vi "MFLI--reader--V3.vi"() -> ()   [LabVIEW 2018]
uses:
  publisher action.ctl
  MFLI frontend action.ctl
  mfli reader event.ctl
panel:
  in  "stop  !":bool
  in  "start  !":bool
  in  "set amp! :m":bool
  in  "amplitude (V)":dbl=0.01
  in  "all":enum32{"all"}(tab)
  out "read Voltage (V)":cdb=-2.6434832298996336e-07+7.155979121852138e-05i format="%#10_10f"
  in  "read status":bool
  out "read Voltage X (V)":dbl=-2.6434832298996336e-07 format="%#11_11f"
  out "read Voltage Y (V)":dbl=7.155979121852138e-05 format="%#11_11f"
  in  "delay-read (msec)":i64=200
  out "zi freq (Hz)":dbl=99999.99999990905 format="%-#.3f"
  in  "MFLI Address":string="http://mf-dev4307.local:8004"
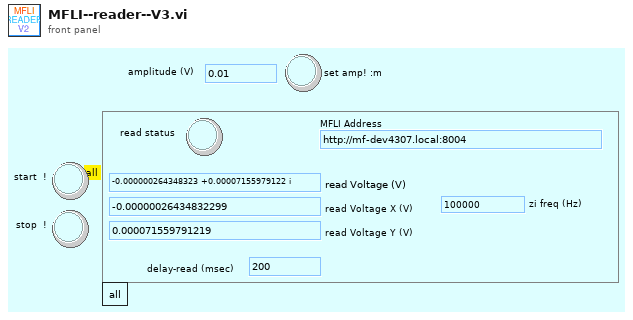
[diagram p1: front panel]
types:
  T1 = typedef "MFLI frontend action.ctl" = enum16{"read", "writeread", "open", "close", "write"}
  T2 = typedef "mfli reader event.ctl" = enum16{"start", "stop"}
  T3 = typedef "publisher action.ctl" = enum16{"set", "get", "init", "check"}
  T4 = typedef "Zurich Instruments LabOne.lvlib/ziTypeHandle.ctl" = cluster{"handleValid":bool, "Conn":u64, "Path Prefix":string, "Handle":u64, "Connected":bool, "Clockbase(s)":dbl}
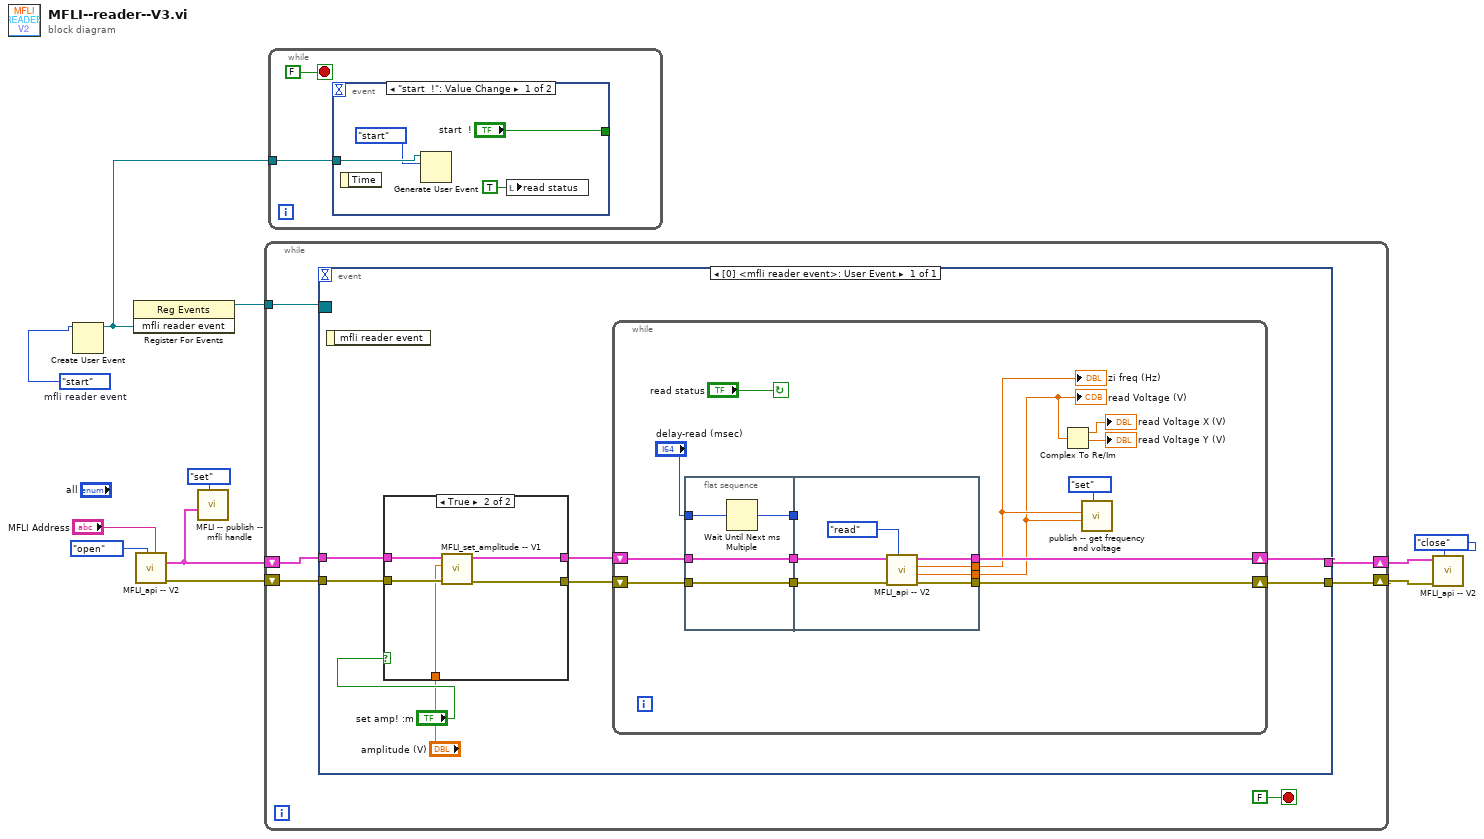
[diagram p0: block diagram]
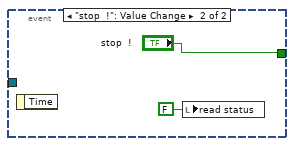
[diagram p3: hidden frame]
diagram:
  w7 = mfli_reader_event."start"  # mfli reader event
  n1 = Create User Event(user event datatype=w7) -> (user event=w6:refnum<user-event>)  [unwired: 1 in, 1 out]
  n2 = register-events(w6) -> (reference out=w8:refnum<event-registration>)  [unwired: 2 in, 1 out]
  n3 = call "MFLI_api -- V2.vi"("MFLI Address"="MFLI Address", "MFLI frontend action"=MFLI_frontend_action."open") -> ("Error Out"=w1:errorcluster, "Handle Out"=w2:T4)  [unwired: 6 in, 2 out]
  n4 = call "MFLI -- publish -- mfli handle.vi"("publisher action"=publisher_action."set", "Handle IN"=w2) -> ()  [unwired: 9 in, 1 out]
  n5 = while {
    tunnel: w8 -> [w17]
    shift-right: [w15] -> w3
    shift-left: w2 -> [w14]
    shift-right: [w16] -> w4
    shift-left: w1 -> [w13]
    stop <- FALSE stop-if-true
    n6 = event shown="[0] <mfli reader event>: User Event" {
      selector: w17 -> [_]
      dyn-events: _ -> [_]
      timeout: _ -> [_]
      tunnel: w14 -> [w24]
      tunnel: w13 -> [w22]
      tunnel: [w19] -> w16
      tunnel: [w18] -> w15
      event User Event {
        n7 = event-data() -> ()  [unwired: 1 in, 1 out]
        n8 = case shown="True" "set amp! :m" {
          tunnel: w24 -> [w27 w32]
          tunnel: [w27 w31] -> w23
          tunnel: w22 -> [w26 w30]
          tunnel: [w26 w29] -> w21
          tunnel: "amplitude (V)" -> [_ w28]
          frame False {
          }
          frame True {
            n9 = call "MFLI_set_amplitude -- V1.vi"("Error In"=w30, "Amp in (V)"=w28, "Handle In"=w32) -> ("Error Out"=w29:errorcluster, "Handle Out"=w31:T4)  [unwired: 5 in, 2 out]
          }
        }
        n10 = while {
          shift-right: [w45] -> w19
          shift-left: w21 -> [w46]
          shift-right: [w43] -> w18
          shift-left: w23 -> [w44]
          stop <- "read status" continue-if-true
          n11 = flat-sequence {
            tunnel: [w50] -> w41
            tunnel: "delay-read (msec)" -> [w49]
            tunnel: [w48] -> w40
            tunnel: w46 -> [w48]
            tunnel: w44 -> [w47]
            tunnel: [w47] -> w39
            tunnel: w41 -> [_]
            tunnel: [w55] -> w33
            tunnel: [w54] -> w34
            tunnel: w40 -> [w57]
            tunnel: [w56] -> w45
            tunnel: w39 -> [w53]
            tunnel: [w52] -> w43
            frame #0 {
              n12 = Wait Until Next ms Multiple(millisecond multiple=w49) -> (millisecond timer value=w50:u32)
            }
            frame #1 {
              n13 = call "MFLI_api -- V2.vi"("MFLI frontend action"=MFLI_frontend_action."read", "Error In"=w57, "Handle In"=w53) -> ("Error Out"=w56:errorcluster, "z out (V)"=w55:cdb, "Freq out (Hz)"=w54:dbl, "Handle Out"=w52:T4)  [unwired: 5 in]
            }
          }
          n14 = Complex To Re/Im(x + iy=w33) -> (x=→"read Voltage X (V)":dbl, y=→"read Voltage Y (V)":dbl)
          n15 = call "publish -- get frequency and voltage.vi"("publisher action"=publisher_action."set", "Voltage IN (V)"=w33, "freq IN (Hz)"=w34) -> ()  [unwired: 6 in, 3 out]
          "read Voltage (V)" <- w33
          "zi freq (Hz)" <- w34
        }
      }
    }
  }
  n16 = while {
    tunnel: w6 -> [w59]
    stop <- FALSE stop-if-true
    n17 = event shown="[0] \"start  !\": Value Change" {
      selector: _ -> [_ _]
      dyn-events: _ -> [_ _]
      timeout: _ -> [_ _]
      tunnel: ["start  !" "stop  !"] -> _
      tunnel: w59 -> [w61 _]
      event "start  !": Value Change {
        n18 = event-data() -> ()  [unwired: 1 in, 1 out]
        n19 = Generate User Event(user event=w61, event data cluster=mfli_reader_event."start" ("event data")) -> ()  [unwired: 2 in, 2 out]
        n20 = local write "read status"(TRUE ("read status")) -> ()
      }
      event "stop  !": Value Change {
        n21 = event-data() -> ()  [unwired: 1 in, 1 out]
        n22 = local write "read status"(FALSE ("read status")) -> ()
      }
    }
  }
  n23 = call "MFLI_api -- V2.vi"("MFLI frontend action"=MFLI_frontend_action."close", "Error In"=w4, "Handle In"=w3) -> ()  [unwired: 5 in, 4 out]
